vi "unload.vi"(8 "error in (no error)":errorcluster, 11 "interface in":refnum<class "interface.lvclass">=refnum) -> (0 "error out":errorcluster, 3 "interface out":refnum<class "interface.lvclass">)   [LabVIEW 2015, in "functional.lvlib" / "interface.lvclass"]
uses:
  interface.lvclass
  interface.lvclass/interface.ctl
  _controls/event_data.ctl
  _controls/event_command.ctl
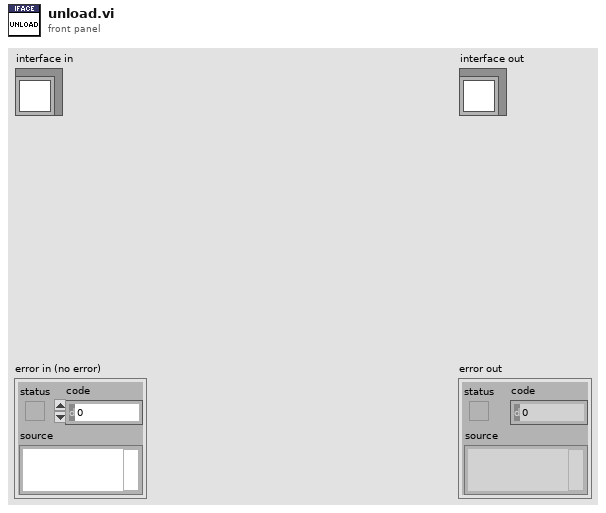
[diagram p1: front panel]
types:
  T1 = typedef "functional.lvlib/interface.lvclass/event_data.ctl" = cluster{"command":T2, "data":variant}
  T2 = typedef "functional.lvlib/interface.lvclass/event_command.ctl" = enum16{"<event_command>", "stop", "<null>"}
  T3 = typedef "functional.lvlib/interface.lvclass/vi_reference.ctl" = refnum<vi>
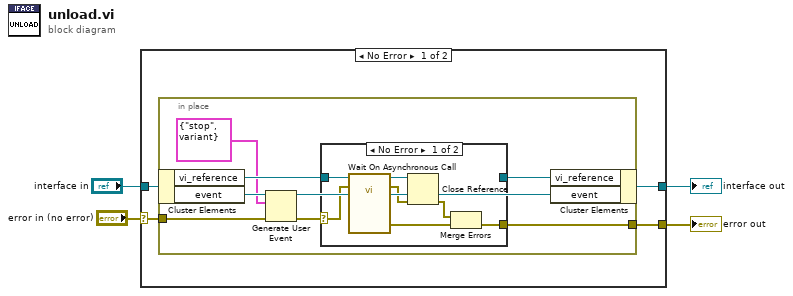
[diagram p0: block diagram]
diagram:
  n1 = case shown="No Error" "error in (no error)" {
    selector: "error in (no error)" -> [w5 w27]
    tunnel: [w8 w27] -> w1
    tunnel: [w6 w26] -> w2
    tunnel: "interface in" -> [w7 w26]
    frame No Error {
      n2 = in-place {
        in-place-border: w5 -> [w11]
        in-place-border: [w15] -> w8
        n3 = in-place-cluster #1(w7) -> ("vi_reference"=w16:T3, "event"=w14:refnum<user-event>)
        n4 = Generate User Event(user event=w14, event data cluster=T1 {"command"=enum."stop", "data"=variant} ("event data"), error in=w11) -> (user event out=w12:refnum<user-event>, error out=w10:errorcluster)  [unwired: 1 in]
        n5 = case shown="No Error" w10 {
          selector: w10 -> [w17 w25]
          tunnel: w16 -> [w23 w24]
          tunnel: [w18 w25] -> w15
          tunnel: [_ w24] -> w9
          frame No Error {
            n6 = call-by-ref "Wait On Asynchronous Call"(reference=w23, error in=w17) -> (reference out=w22:T3, error out=w21:errorcluster, 0:"error out"=w19:errorcluster)  [unwired: 11 in]
            n7 = Close Reference(reference=w22, error in (no error)=w21) -> (error out=w20:errorcluster)
            n8 = Merge Errors(w20, w19) -> (w18:errorcluster)
          }
          frame Error {
          }
        }
        n9 = in-place-cluster #1("vi_reference"=w9, "event"=w12) -> (w6:refnum<class "interface.lvclass">)
      }
    }
    frame Error {
    }
  }
  "error out" <- w1
  "interface out" <- w2
